vi "dfd_DA Global Para.vi"() -> ()   [LabVIEW 2017, in "NI_DigFilter_CodeGen.lvlib"]
uses:
  <vilib>/addons/Digital Filter Design/NI_DigFilter_CodeGen.lvlib
panel:
  in  "Resource Threshhold":u32=8000
  in  "Max tap count":u32=300
  in  "Min coeff wl":u32=4
  in  "Min input wl":u32=1
  in  "Max coeff wl":u32=32
  in  "Max factor":i8=8
  in  "Max # of channels":i8=8
  in  "Max input wl":u32=32
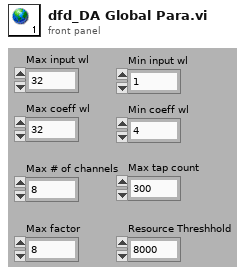
[diagram p1: front panel]
diagram:
